vi "Into Tree Control Items.vi"(7 "Preserve Insertion Order? (F)":bool, 10 "Paths Set":set{string}(c389), 11 "Tree Map In":T1) -> (3 "Tree Control Item":T2(array[cluster]))   [LabVIEW 2020, in "Tree Map.lvlib"]
doc: "Helper function for converting the Tree Map elements into Tree Control Items. If you would like to unflatten the data in a different way, modify glyps or change the Tree Control Items array, you can copy and modify the code of this VI or make your changes after or before it runs.\n\n<b>Author:</b> Piotr Kruczkowski <PrimaryKey>\n<b>License:</b> NewBSD\n\nCopyright (c) 2019, National Instruments\nAll rights reserved.\n\nRedistribution and use in source and binary forms, with or without\nmodification, are permitted provided that the following conditions are met:\n1. Redistributions of source code must retain the above copyright\n notice, this list of conditions and the following disclaimer.\n2. Redistributions in binary form must reproduce the above copyright\n notice, this list of conditions and the following disclaimer in the\n documentation and/or other materials provided with the distribution.\n3. Neither the name of National Instruments nor the\n names of its contributors may be used to endorse or promote products\n derived from this software without specific prior written permission.\n\nTHIS SOFTWARE IS PROVIDED BY National Instruments ''AS IS'' AND ANY\nEXPRESS OR IMPLIED WARRANTIES, INCLUDING, BUT NOT LIMITED TO, THE IMPLIED\nWARRANTIES OF MERCHANTABILITY AND FITNESS FOR A PARTICULAR PURPOSE ARE\nDISCLAIMED. IN NO EVENT SHALL National Instruments BE LIABLE FOR ANY\nDIRECT, INDIRECT, INCIDENTAL, SPECIAL, EXEMPLARY, OR CONSEQUENTIAL DAMAGES\n(INCLUDING, BUT NOT LIMITED TO, PROCUREMENT OF SUBSTITUTE GOODS OR SERVICES;\nLOSS OF USE, DATA, OR PROFITS; OR BUSINESS INTERRUPTION) HOWEVER CAUSED AND\nON ANY THEORY OF LIABILITY, WHETHER IN CONTRACT, STRICT LIABILITY, OR TORT\n(INCLUDING NEGLIGENCE OR OTHERWISE) ARISING IN ANY WAY OUT OF THE USE OF THIS\nSOFTWARE, EVEN IF ADVISED OF THE POSSIBILITY OF SUCH DAMAGE."
uses:
  Tree Map.lvlib
  Tree Map Data.ctl
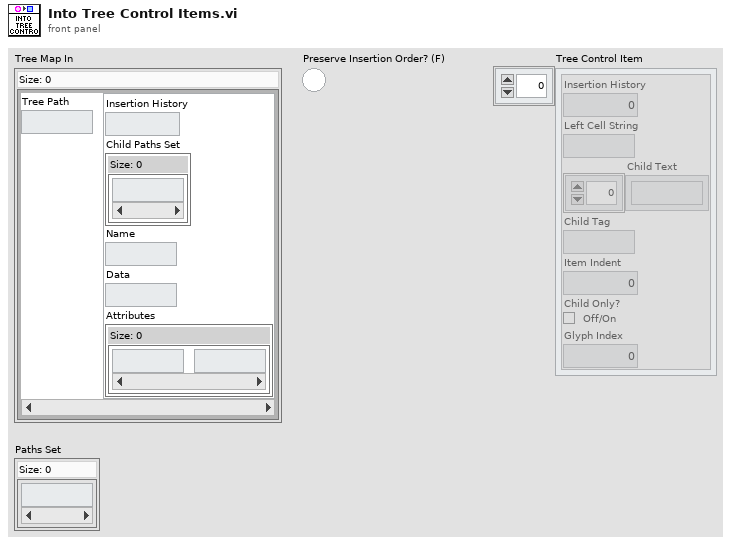
[diagram p1: front panel]
types:
  T1 = typedef "Tree Map.lvlib/Tree Map Data.ctl" = map{string, cluster{"Insertion History":i32, "Child Paths Set":set{string}, "Name":string, "Data":string, "Attributes":map{string, string}}}
  T2 = cluster{"Insertion History":i32, "Left Cell String":string, "Child Text":string[], "Child Tag":string, "Item Indent":i32, "Child Only?":bool, "Glyph Index":i32}[]
  T3 = cluster{"Insertion History":i32, "Left Cell String":string, "Child Text":string[], "Child Tag":string, "Item Indent":i32, "Child Only?":bool, "Glyph Index":i32}
  T4 = cluster{"Insertion History":i32, "Child Paths Set":set{string}, "Name":string, "Data":string, "Attributes":map{string, string}}
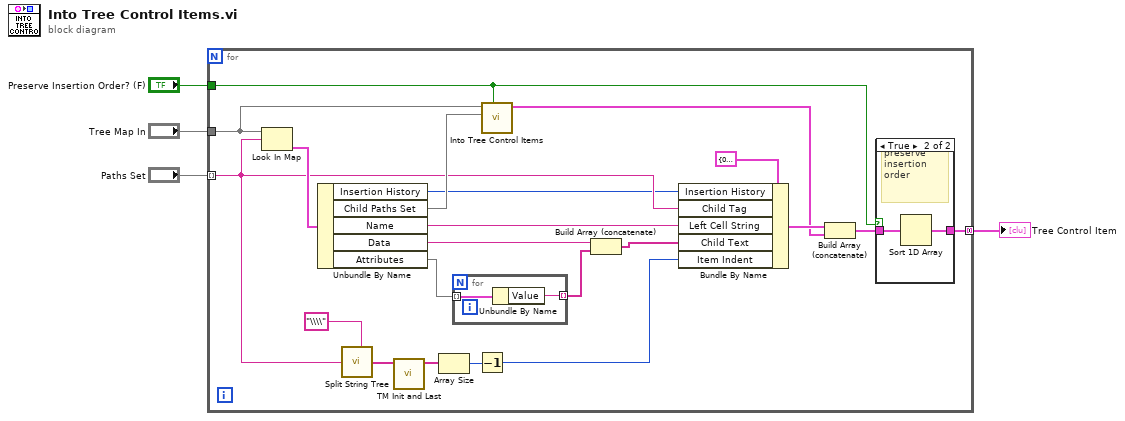
[diagram p0: block diagram]
diagram:
  n1 = for {
    tunnel: "Paths Set" -> [w16] mode=indexing
    tunnel: [w7] -> w2 mode=concatenating
    tunnel: "Tree Map In" -> [w24]
    tunnel: "Preserve Insertion Order? (F)" -> [w5]
    n2 = Look In Map(map=w24, key=w16) -> (value=w25:T4)  [unwired: 1 in, 1 out]
    n3 = Unbundle By Name(w25) -> ("Insertion History"=w6:i32, "Child Paths Set"=w23:set{string}, "Name"=w21:string, "Data"=w12:string, "Attributes"=w15:map{string, string})
    n4 = call "Split String Tree.vi"("Split Pattern"="\\\\", "Input String"=w16) -> ("Split String"=w17:string[])  [unwired: 5 in]
    n5 = call "TM Init and Last.vi"("List"=w17) -> ("Init List"=w19:string[])  [unwired: 9 in, 1 out]
    n6 = Array Size(array=w19) -> (size(s)=w20:i32)
    n7 = for {
      tunnel: w15 -> [w30] mode=indexing
      tunnel: [w29] -> w13 mode=indexing
      n8 = Unbundle By Name(w30) -> ("Value"=w29:string)
    }
    n9 = Decrement(x=w20) -> (x-1=w14:i32)
    n10 = call "Into Tree Control Items.vi"("Preserve Insertion Order? (F)"=w5, "Paths Set"=w23, "Tree Map In"=w24) -> ("Tree Control Item"=w9:T2)  [unwired: 8 in]
    n11 = Build Array (concatenate)(w12, w13) -> (w11:string[])
    n12 = Bundle By Name(cluster=T3 {"Insertion History"=0, "Left Cell String"="", "Child Text"=[], "Child Tag"="", "Item Indent"=0, "Child Only?"=FALSE, "Glyph Index"=0} ("Item"), "Insertion History"=w6, "Child Tag"=w16, "Left Cell String"=w21, "Child Text"=w11, "Item Indent"=w14) -> (w10:T3)
    n13 = Build Array (concatenate)(w10, w9) -> (w8:T2)
    n14 = case shown="True" w5 {
      tunnel: w8 -> [w26 w28]
      tunnel: [w26 w27] -> w7
      frame False {
      }
      frame True {
        # "preserve insertion order"
        n15 = Sort 1D Array(array=w28) -> (sorted array=w27:T2)
      }
    }
  }
  "Tree Control Item" <- w2
